vi "Ibeopaser.vi"(6 "theta":dbl, 8 "Hide Transparent":bool=TRUE, 11 "Sensor [F12]":bool=TRUE) -> (0 "x_sensor":cluster{"idx":i32, "x":dbl, "y":dbl, "h":dbl}, 1 "etc":dbl[][](array[numeric]), 2 "lane":dbl[][](array[numeric]), 3 "obs":dbl[][](array[numeric]), 4 "update":bool)   [LabVIEW 2015]
uses:
  G_LCM.vi
panel:
  out "error IO":errorcluster
  out "dz":dbl
  out "dy":dbl
  out "dx":dbl
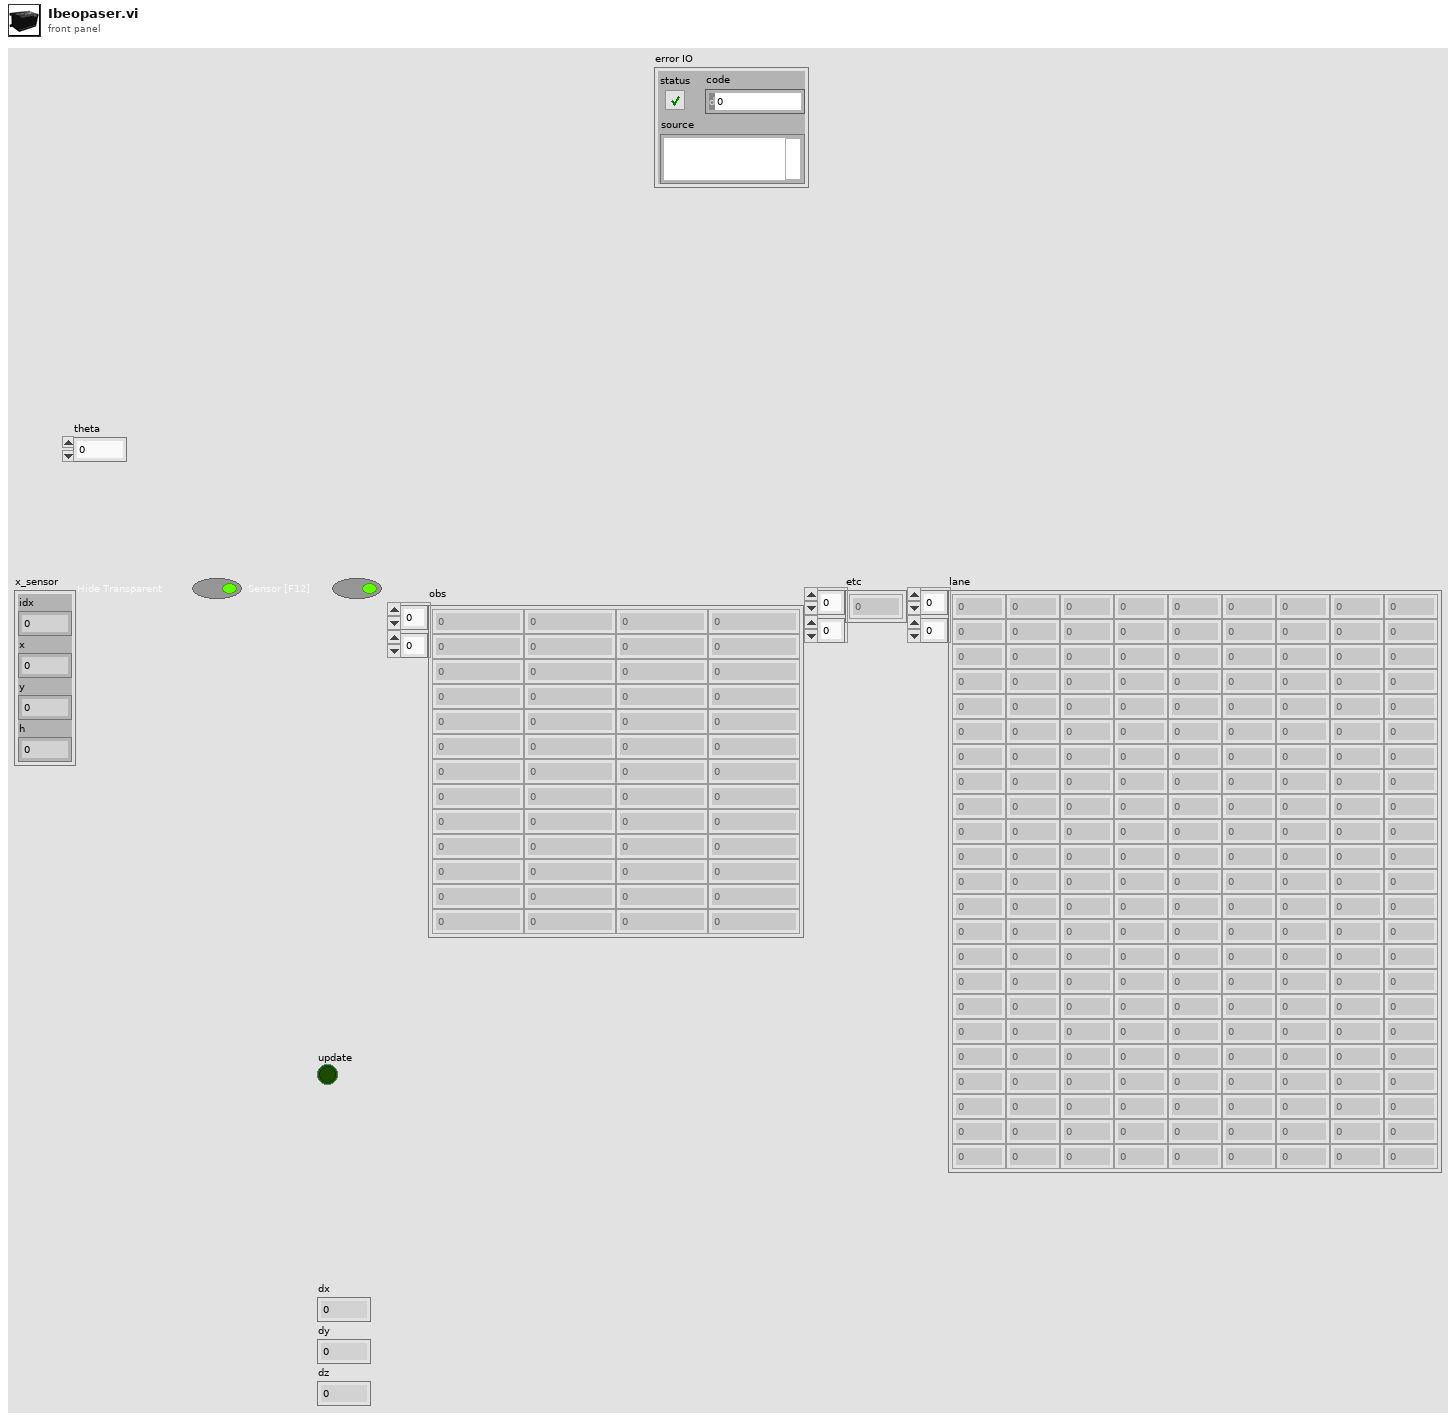
[diagram p1: front panel]
types:
  T1 = cluster{"hash":i64, "sys time":i64, "Header":cluster{"Size of prev messages":u32, "Size of this messages":u32, "Reserved":u8, "DeviceID":u8, "Data type":u16, "NTP time":u64}, "Scan header":cluster{"Scan number":u16, "scanner status":u16, "Sync phase offset":u16, "Scan start time NTP":u64, "Scan end time NTP":u64, "Angle ticks per rotation":u16, "Start angle":dbl, "End angle":dbl, "Scan points":u16, "pos_x":dbl, "pos_y":dbl, "pos_h":dbl, "Mounting position x":dbl, "Mounting position y":dbl, "Mounting position z":dbl, "Reserved":u16}, "Scan points":cluster{"flags":u8, "Echo":u8, "Radial distance":dbl, "Horizontal angle":dbl, "Vertical angle":dbl, "Echo pulse width":u16, "Reserved":u16}[]}
  T2 = cluster{"Scan number":u16, "scanner status":u16, "Sync phase offset":u16, "Scan start time NTP":u64, "Scan end time NTP":u64, "Angle ticks per rotation":u16, "Start angle":dbl, "End angle":dbl, "Scan points":u16, "pos_x":dbl, "pos_y":dbl, "pos_h":dbl, "Mounting position x":dbl, "Mounting position y":dbl, "Mounting position z":dbl, "Reserved":u16}
  T3 = cluster{"flags":u8, "Echo":u8, "Radial distance":dbl, "Horizontal angle":dbl, "Vertical angle":dbl, "Echo pulse width":u16, "Reserved":u16}[]
  T4 = cluster{i16, dbl, dbl, dbl, dbl, "Echo pulse width":u16}[]
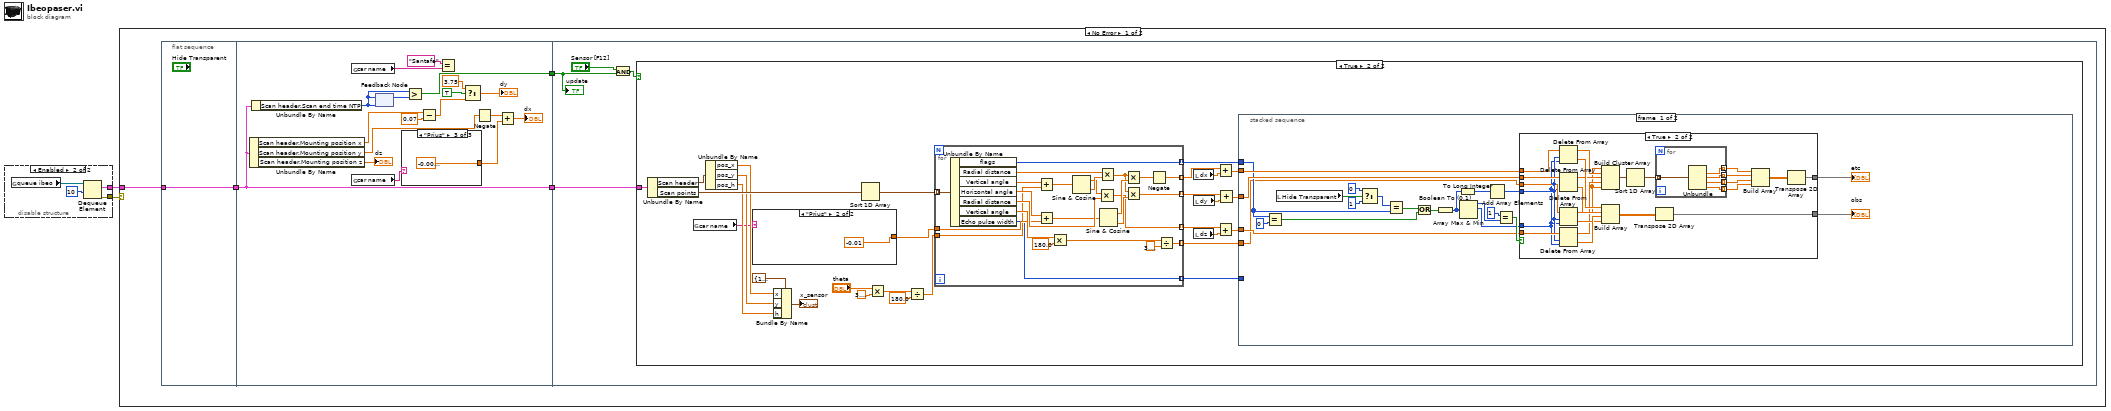
[diagram p0: block diagram]
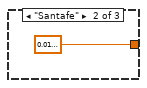
[diagram p3: hidden frame]
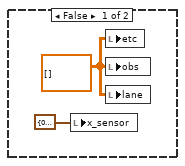
[diagram p4: hidden frame]
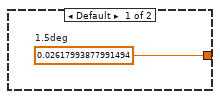
[diagram p5: hidden frame]
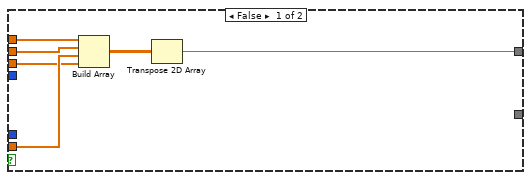
[diagram p6: hidden frame]
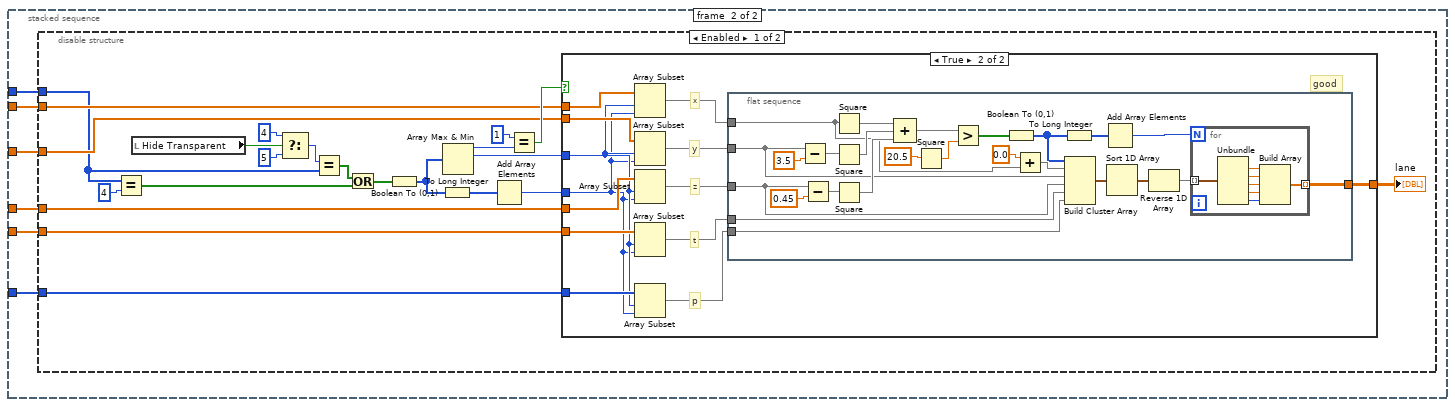
[diagram p7: hidden frame]
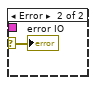
[diagram p10: hidden frame]
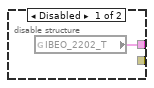
[diagram p11: hidden frame]
diagram:
  n1 = disable-structure shown="Enabled" {
    disable-tunnel: [w3 w6] -> w1
    disable-tunnel: [_ w4] -> w2
    frame Disabled {
      n2 = global read "G_LCM.vi" "IBEO_2202_T"() -> (w3:T1)
    }
    frame Enabled {
      n3 = global read "G_LCM.vi" "queue ibeo"() -> (w7:refnum<queue>)
      n4 = Dequeue Element(queue=w7, timeout in ms (-1)=10) -> (element=w6:T1, error out=w4:errorcluster)  [unwired: 1 in, 2 out]
    }
  }
  n5 = case shown="No Error" w2 {
    selector: w2 -> [_ w224]
    tunnel: w1 -> [w8 _]
    frame No Error {
      n6 = flat-sequence {
        tunnel: [w12] -> w11
        tunnel: w8 -> [w12]
        tunnel: [w30] -> w10
        tunnel: w11 -> [w25]
        tunnel: [w25] -> w9
        tunnel: w10 -> [w35]
        tunnel: w9 -> [w33]
        frame #0 {
        }
        frame #1 {
          n7 = Unbundle By Name(w25) -> ("Scan header.Mounting position x"=w28:dbl, "Scan header.Mounting position y"=w26:dbl, "Scan header.Mounting position z"=→"dz":dbl)
          n8 = Unbundle By Name(w25) -> ("Scan header.Scan end time NTP"=w23:u64)
          n9 = global read "G_LCM.vi" "car name"() -> (w22:string)
          n10 = global read "G_LCM.vi" "car name"() -> (w14:string)
          n11 = feedback #1(w23) -> (w24:u64)
          n12 = feedback-in #1(w23) -> ()
          n13 = case shown="\"Prius\"" w14 {
            tunnel: [_ 0.019999999999999997 ("Numeric") -0.009999999999999997 ("Numeric")] -> w13
            frame Default {
            }
            frame "Santafe" {
            }
            frame "Prius" {
            }
          }
          n14 = Greater?(x=w23, y=w24) -> (0:w30:bool)
          n15 = Subtract(x=w28, y=0.07) -> (x-y=w19:dbl)
          n16 = Equal?(x="Santafe", y=w22) -> ()  [unwired: 1 out]
          n17 = Select(t=3.75 ("dy"), s=TRUE, f=w19) -> (s? t:f=→"dy":dbl)
          n18 = Negate(x=w26) -> (-x=w16:dbl)
          n19 = Add(x=w16, y=w13) -> (x+y=→"dx":dbl)
        }
        frame #2 {
          n20 = And(x="Sensor [F12]", y=w35) -> (x .and. y?=w34:bool)
          n21 = case shown="True" w34 {
            tunnel: w33 -> [_ w53]
            frame False {
              w38 = dbl[][] [] ("lane")
              n22 = local write "x_sensor"(cluster{"idx":i32, "x":dbl, "y":dbl, "h":dbl} {"idx"=0, "x"=0.0, "y"=0.0, "h"=0.0} ("x_sensor")) -> ()
              n23 = local write "etc"(w38) -> ()
              n24 = local write "obs"(w38) -> ()
              n25 = local write "lane"(w38) -> ()
            }
            frame True {
              n26 = Unbundle By Name(w53) -> ("Scan header"=w58:T2, "Scan points"=w62:T3)
              n27 = global read "G_LCM.vi" "car name"() -> (w40:string)
              n28 = Unbundle By Name(w58) -> ("pos_x"=w56:dbl, "pos_y"=w55:dbl, "pos_h"=w57:dbl)
              n29 = case shown="\"Prius\"" w40 {
                tunnel: [w67 -0.01 ("1.5deg")] -> w39
                frame Default {
                  w67 = 0.02617993877991494  # 1.5deg
                }
                frame "Prius" {
                }
              }
              n30 = Bundle By Name(cluster=cluster{"idx":i32, "x":dbl, "y":dbl, "h":dbl} {"idx"=1, "x"=0.0, "y"=0.0, "h"=0.0} ("xsensor"), "x"=w56, "y"=w55, "h"=w57) -> (→"x_sensor":cluster{"idx":i32, "x":dbl, "y":dbl, "h":dbl})
              n31 = Sort 1D Array(array=w62) -> (sorted array=w61:T3)
              n32 = Multiply(x="theta", y=3.141592653589793) -> (x*y=w46:dbl)
              n33 = Divide(x=w46, y=180.0) -> (x/y=w42:dbl)
              n34 = for {
                tunnel: w61 -> [w93] mode=indexing
                tunnel: w39 -> [w79]
                tunnel: [w77] -> w66 mode=indexing
                tunnel: [w76] -> w51 mode=indexing
                tunnel: [w75] -> w50 mode=indexing
                tunnel: [w74] -> w47 mode=indexing
                tunnel: [w73] -> w60 mode=indexing
                tunnel: [w72] -> w59 mode=indexing
                tunnel: w42 -> [w69]
                n35 = Unbundle By Name(w93) -> ("flags"=w77:u8, "Radial distance"=w87:dbl, "Vertical angle"=w71:dbl, "Horizontal angle"=w80:dbl, "Radial distance"=w81:dbl, "Vertical angle"=w85:dbl, "Echo pulse width"=w72:u16)
                n36 = Add(x=w71, y=w69) -> (x+y=w70:dbl)
                n37 = Add(x=w80, y=w79) -> (x+y=w78:dbl)
                n38 = Multiply(x=w85, y=180.0) -> (x*y=w84:dbl)
                n39 = Sine & Cosine(0:w70) -> (1:w86:dbl, 2:w88:dbl)
                n40 = Multiply(x=w86, y=w81) -> (x*y=w74:dbl)
                n41 = Multiply(x=w87, y=w88) -> (x*y=w90:dbl)
                n42 = Sine & Cosine(0:w78) -> (1:w92:dbl, 2:w91:dbl)
                n43 = Multiply(x=w90, y=w92) -> (x*y=w89:dbl)
                n44 = Multiply(x=w90, y=w91) -> (x*y=w75:dbl)
                n45 = Negate(x=w89) -> (-x=w76:dbl)
                n46 = Divide(x=w84, y=3.141592653589793) -> (x/y=w73:dbl)
              }
              n47 = local read "dx"() -> (w52:dbl)
              n48 = local read "dy"() -> (w49:dbl)
              n49 = local read "dz"() -> (w48:dbl)
              n50 = Add(x=w51, y=w52) -> (x+y=w65:dbl[])
              n51 = Add(x=w47, y=w48) -> (x+y=w63:dbl[])
              n52 = Add(x=w50, y=w49) -> (x+y=w64:dbl[])
              n53 = stacked-sequence {
                tunnel: w66 -> [w107 w153]
                tunnel: w65 -> [w110 w156]
                tunnel: w64 -> [w109 w155]
                tunnel: w63 -> [w108 w154]
                tunnel: w60 -> [w98 w152]
                tunnel: w59 -> [_ w151]
                frame #0 {
                  n54 = Equal?(x=w107, y=u8 0) -> (x = y?=w105:bool[])
                  n55 = local read "Hide Transparent"() -> (w102:bool)
                  n56 = Select(t=u8 0, s=w102, f=u8 1) -> (s? t:f=w99:u8)
                  n57 = Equal?(x=w99, y=w107) -> (x = y?=w104:bool[])
                  n58 = Or(x=w104, y=w105) -> (x .or. y?=w103:bool[])
                  n59 = Boolean To (0,1)(Boolean=w103) -> (0, 1=w97:i16[])
                  n60 = To Long Integer(number=w97) -> (32bit integer=w96:i32[])
                  n61 = Array Max & Min(array=w97) -> (max value=w115:i16, max index (indices)=w111:i32)  [unwired: 2 out]
                  n62 = Add Array Elements(numeric array=w96) -> (sum=w112:i32)
                  n63 = Equal?(x=i16 1, y=w115) -> (x = y?=w113:bool)
                  n64 = case shown="True" w113 {
                    tunnel: w112 -> [_ w134]
                    tunnel: w111 -> [_ w133]
                    tunnel: w110 -> [w121 w137]
                    tunnel: w109 -> [w120 w145]
                    tunnel: [_ w138] -> w95
                    tunnel: w108 -> [w119 w143]
                    tunnel: w98 -> [w118 w141]
                    tunnel: [w116 w135] -> w94
                    frame False {
                      n65 = Build Array(w121, w120, w119, w118) -> (w117:dbl[][])
                      n66 = Transpose 2D Array(2D array=w117) -> (transposed array=w116:dbl[][])
                    }
                    frame True {
                      n67 = Delete From Array(array=w137, length=w134, index=w133) -> (deleted portion=w139:dbl[], array with subset deleted=w131:dbl[])
                      n68 = Delete From Array(array=w145, length=w134, index=w133) -> (deleted portion=w144:dbl[], array with subset deleted=w130:dbl[])
                      n69 = Delete From Array(array=w141, length=w134, index=w133) -> (deleted portion=w140:dbl[], array with subset deleted=w128:dbl[])
                      n70 = Delete From Array(array=w143, length=w134, index=w133) -> (deleted portion=w142:dbl[], array with subset deleted=w129:dbl[])
                      n71 = Build Cluster Array(w128, w131, w130, w129, w128) -> (w127:cluster{dbl, dbl, dbl, dbl, dbl}[])
                      n72 = Build Array(w139, w144, w142, w140) -> (w132:dbl[][])
                      n73 = Sort 1D Array(array=w127) -> (sorted array=w126:cluster{dbl, dbl, dbl, dbl, dbl}[])
                      n74 = for {
                        tunnel: w126 -> [w150] mode=indexing
                        tunnel: [w149] -> w125 mode=indexing
                        tunnel: [w148] -> w124 mode=indexing
                        tunnel: [w147] -> w123 mode=indexing
                        tunnel: [w146] -> w122 mode=indexing
                        n75 = Unbundle(w150) -> (w149:dbl, w148:dbl, w147:dbl, w146:dbl)  [unwired: 1 out]
                      }
                      n76 = Transpose 2D Array(2D array=w132) -> (transposed array=w138:dbl[][])
                      n77 = Build Array(w125, w124, w123, w122) -> (w136:dbl[][])
                      n78 = Transpose 2D Array(2D array=w136) -> (transposed array=w135:dbl[][])
                    }
                  }
                  "obs" <- w95
                  "etc" <- w94
                }
                frame #1 {
                  n79 = disable-structure shown="Enabled" {
                    disable-tunnel: w156 -> [w173 _]
                    disable-tunnel: w155 -> [w172 _]
                    disable-tunnel: w154 -> [w171 _]
                    disable-tunnel: w153 -> [w170 _]
                    disable-tunnel: w152 -> [w160 _]
                    disable-tunnel: w151 -> [w159 _]
                    frame Enabled {
                      n80 = Equal?(x=w170, y=u8 4) -> (x = y?=w168:bool[])
                      n81 = local read "Hide Transparent"() -> (w165:bool)
                      n82 = Select(t=u8 4, s=w165, f=u8 5) -> (s? t:f=w162:u8)
                      n83 = Equal?(x=w162, y=w170) -> (x = y?=w167:bool[])
                      n84 = Or(x=w167, y=w168) -> (x .or. y?=w166:bool[])
                      n85 = Boolean To (0,1)(Boolean=w166) -> (0, 1=w157:i16[])
                      n86 = To Long Integer(number=w157) -> (32bit integer=w158:i32[])
                      n87 = Array Max & Min(array=w157) -> (max value=w178:i16, max index (indices)=w174:i32)  [unwired: 2 out]
                      n88 = Add Array Elements(numeric array=w158) -> (sum=w175:i32)
                      n89 = Equal?(x=i16 1, y=w178) -> (x = y?=w176:bool)
                      n90 = case shown="True" w176 {
                        tunnel: w175 -> [_ w185]
                        tunnel: w174 -> [_ w186]
                        tunnel: w173 -> [_ w191]
                        tunnel: w172 -> [_ w190]
                        tunnel: [_ w179] -> w161
                        tunnel: w171 -> [_ w189]
                        tunnel: w160 -> [_ w188]
                        tunnel: w159 -> [_ w187]
                        frame False {
                        }
                        frame True {
                          # "good"
                          # "p"
                          # "t"
                          # "z"
                          # "y"
                          # "x"
                          n91 = Array Subset(array=w191, index=w186, length=w185) -> (w180:dbl[])
                          n92 = Array Subset(array=w190, index=w186, length=w185) -> (w184:dbl[])
                          n93 = Array Subset(array=w189, index=w186, length=w185) -> (w183:dbl[])
                          n94 = Array Subset(array=w188, index=w186, length=w185) -> (w182:dbl[])
                          n95 = Array Subset(array=w187, index=w186, length=w185) -> (w181:u16[])
                          n96 = flat-sequence {
                            tunnel: w184 -> [w206]
                            tunnel: w183 -> [w205]
                            tunnel: w182 -> [w193]
                            tunnel: w181 -> [w204]
                            tunnel: [w194] -> w179
                            tunnel: w180 -> [w200]
                            frame #0 {
                              n97 = Subtract(x=w206, y=3.5) -> (x-y=w215:dbl[])
                              n98 = Subtract(x=w205, y=0.45) -> (x-y=w216:dbl[])
                              n99 = Square(x=w200) -> (x^2=w210:dbl[])
                              n100 = Square(x=w215) -> (x^2=w211:dbl[])
                              n101 = Square(x=w216) -> (x^2=w212:dbl[])
                              n102 = Compound Arithmetic op=ADD(w210, w211, w212) -> (w209:dbl[])
                              n103 = Square(x=20.5 ("R 2")) -> (x^2=w207:dbl)
                              n104 = Greater?(x=w209, y=w207) -> (0:w192:bool[])
                              n105 = Boolean To (0,1)(Boolean=w192) -> (0, 1=w196:i16[])
                              n106 = Add(x=0.0, y=w200) -> (x+y=w199:dbl[])
                              n107 = To Long Integer(number=w196) -> (32bit integer=w195:i32[])
                              n108 = Build Cluster Array(w196, w199, w206, w205, w193, w204) -> (w203:T4)
                              n109 = Add Array Elements(numeric array=w195) -> (sum=w197:i32)
                              n110 = Sort 1D Array(array=w203) -> (sorted array=w202:T4)
                              n111 = Reverse 1D Array(array=w202) -> (reversed array=w201:T4)
                              n112 = for {
                                N: w197 -> [_]
                                tunnel: w201 -> [w223] mode=indexing
                                tunnel: [w217] -> w194 mode=indexing
                                n113 = Unbundle(w223) -> (w222:dbl, w221:dbl, w220:dbl, w219:dbl, "Echo pulse width"=w218:u16)  [unwired: 1 out]
                                n114 = Build Array(w222, w221, w220, w219, w218) -> (w217:dbl[])
                              }
                            }
                          }
                        }
                      }
                      "lane" <- w161
                    }
                    frame Disabled {
                    }
                  }
                }
              }
            }
          }
          "update" <- w35
        }
      }
    }
    frame Error {
      "error IO" <- w224
    }
  }
